vi "TENMA 72-2xxx get Iout, oneshot.vi"(0 "Port":refnum<visa-resource-name>) -> (1 "Iout (A)":sgl=nan format="%_4g", 2 "error out":errorcluster)   [LabVIEW 2018]
uses:
  <vilib>/Instr/_visa.llb/VISA Open Access Mode.ctl
  ctls/TENMA 72-2xxx commands.ctl
panel:
  # "PN 13/04/18"
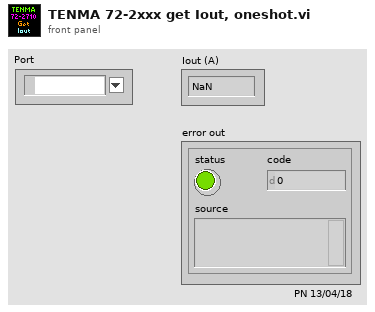
[diagram p1: front panel]
types:
  T1 = typedef "TENMA 72-2xxx commands.ctl" = string
  T2 = typedef "VISA Open Access Mode.ctl" = u32
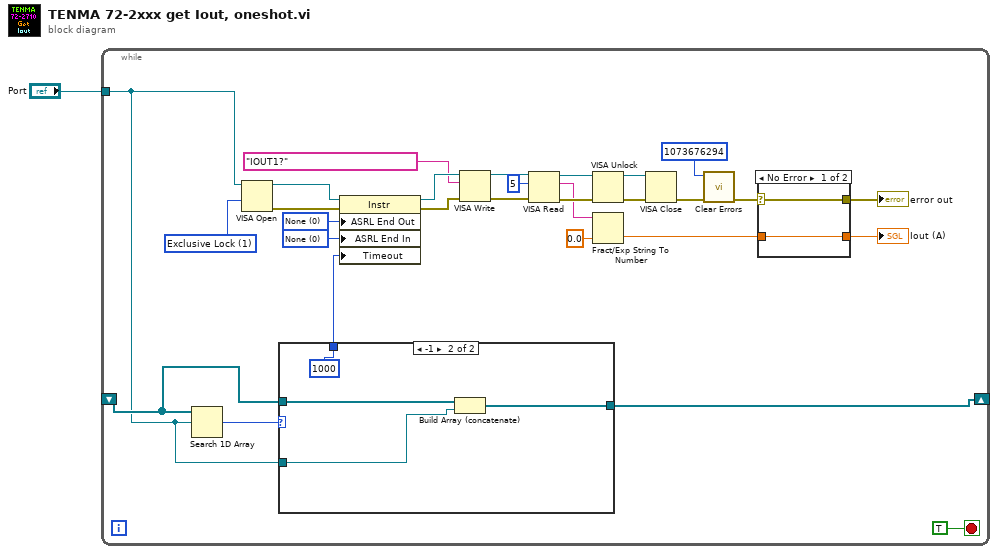
[diagram p0: block diagram]
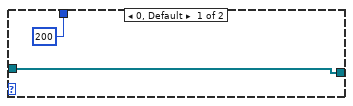
[diagram p2: hidden frame]
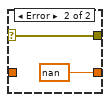
[diagram p3: hidden frame]
diagram:
  n1 = while {
    tunnel: "Port" -> [w5]
    shift-right: [w4] -> _
    shift-left: _ -> [w6]
    stop <- TRUE stop-if-true
    w19 = u16 0 items=["None", "Last Bit", "TermChar"] ("Serial Settings:End Mode for Reads")
    w20 = u16 0 items=["None", "Last Bit", "TermChar", "Break"] ("Serial Settings:End Mode for Writes")
    w30 = T2 1 items=["VISA Defaults"=0, "Exclusive Lock"=1, "Load Configured Settings"=4] ("Access Mode")
    n2 = Search 1D Array(1D array=w6, element=w5) -> (index of element=w7:i32)  [unwired: 1 in]
    n3 = VISA Open(access mode=w30, VISA resource name=w5) -> (VISA resource name=w24:refnum<visa-resource-name>, error out=w22:errorcluster)  [unwired: 3 in]
    n4 = case shown="-1" w7 {
      tunnel: w6 -> [w32 w36]
      tunnel: w5 -> [_ w35]
      tunnel: [w32 w34] -> w4
      tunnel: [u32 200 ("General Settings:Timeout Value") u32 1000 ("General Settings:Timeout Value")] -> w3
      frame 0, Default {
      }
      frame -1 {
        n5 = Build Array (concatenate)(w36, w35) -> (w34:refnum<visa-resource-name>[])
      }
    }
    n6 = property class="Instr"(reference=w24, error in=w22, "ASRL End Out"=w20, "ASRL End In"=w19, "Timeout"=w3) -> (reference out=w23:refnum<visa-resource-name>, error out=w21:errorcluster)
    n7 = VISA Write(VISA resource name=w23, write buffer=T1 "IOUT1?" ("Command"), error in (no error)=w21) -> (VISA resource name out=w17:refnum<visa-resource-name>, error out=w16:errorcluster)  [unwired: 1 out]
    n8 = VISA Read(VISA resource name=w17, byte count=u32 5, error in (no error)=w16) -> (VISA resource name out=w25:refnum<visa-resource-name>, read buffer=w14:string, error out=w26:errorcluster)  [unwired: 1 out]
    n9 = VISA Unlock(8:w26, 11:w25) -> (0:w29:errorcluster, 3:w28:refnum<visa-resource-name>)
    n10 = Fract/Exp String To Number(string=w14, default (0 dbl)=sgl 0.0 ("default (0 DBL)")) -> (number=w8:sgl)  [unwired: 2 in, 1 out]
    n11 = VISA Close(VISA resource name=w28, error in (no error)=w29) -> (error out=w27:errorcluster)
    n12 = call <vilib>:"Clear Errors.vi"("error in (no error)"=w27, "specific error code to clear (0: all)"=1073676294) -> ("error out"=w11:errorcluster)  [unwired: 4 in, 1 out]
    n13 = case shown="No Error" w11 {
      selector: w11 -> [w38 w39]
      tunnel: [w38 w39] -> w10
      tunnel: [w37 sgl nan] -> w9
      tunnel: w8 -> [w37 _]
      frame No Error {
      }
      frame Error {
      }
    }
    "error out" <- w10
    "Iout (A)" <- w9
  }
